vi "CMD_FIT.vi"(6 "Gantry in":refnum<class "Gantry Class.lvclass">, 8 "error in (no error)":errorcluster, 10 "Arguments":string[](array[string]), 11 "gScript Interpreter in":refnum<class "gScript Interpreter.lvclass">) -> (0 "error out":errorcluster, 3 "gScript Interpreter out":refnum<class "gScript Interpreter.lvclass">, 4 "Gantry out":refnum<class "Gantry Class.lvclass">)   [LabVIEW 2017, in "gScript Interpreter.lvclass"]
uses:
  gScript Interpreter.lvclass
  Shared Components/Gantry Class/Gantry Class.lvclass
  Shared Components/Vec3d Class/Vec3d Class.lvclass
  Shared Components/FlexWorktable/FlexWorktable.lvclass
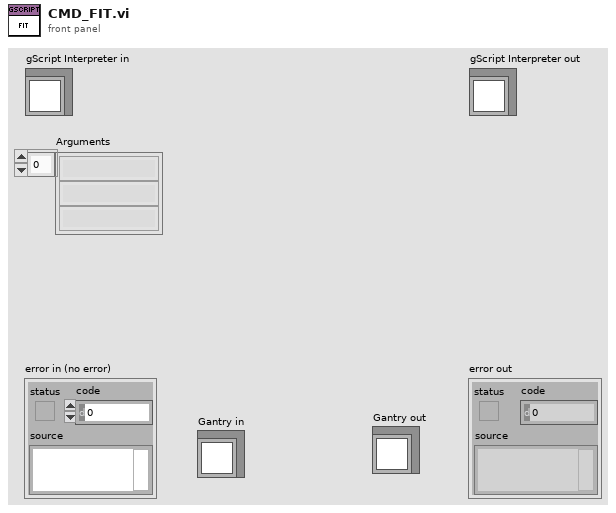
[diagram p1: front panel]
types:
  T1 = cluster{"fiducial location":refnum<class "Vec3d Class.lvclass">, "fiducial name":string}
  T2 = cluster{"Feature Coordinates":refnum<class "Vec3d Class.lvclass">, "Feature Name":string}[]
  T3 = typedef "Memory Cell.ctl" = cluster{"type":T4, "x":dbl, "y":dbl, "z":dbl, "w":dbl}
  T4 = typedef "Memory Cell Type Enum.ctl" = enum16{"integer", "float", "vector", "rotation"}
  T5 = cluster{"fiducial location":refnum<class "Vec3d Class.lvclass">, "fiducial name":string}[]
  T6 = typedef "Position_Orientation.ctl" = cluster{"Center":refnum<class "Vec3d Class.lvclass">, "Orientation":refnum<class "Orient3d Class.lvclass">}
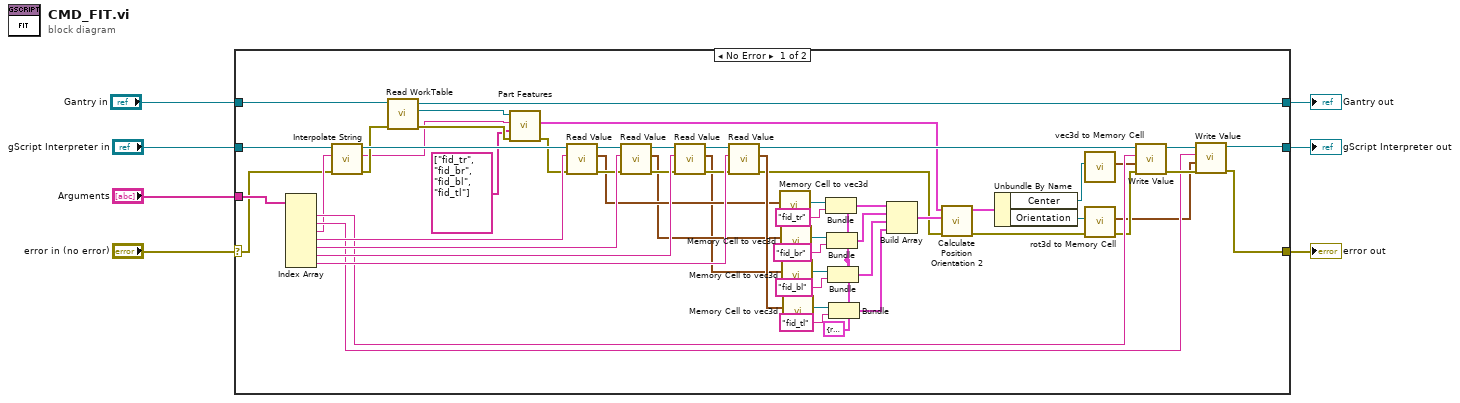
[diagram p0: block diagram]
diagram:
  n1 = case shown="No Error" "error in (no error)" {
    selector: "error in (no error)" -> [w16 w66]
    tunnel: [w19 w66] -> w6
    tunnel: [w20 w65] -> w4
    tunnel: "gScript Interpreter in" -> [w17 w65]
    tunnel: "Arguments" -> [w63 _]
    tunnel: "Gantry in" -> [w62 w64]
    tunnel: [w61 w64] -> w1
    frame No Error {
      w41 = T1 {"fiducial location"=refnum, "fiducial name"=""} ("fiducial with name")
      n2 = Index Array(array=w63) -> (element #1=w29:string, element #2=w23:string, element #3=w18:string, element #4=w60:string, element #5=w59:string, element #6=w58:string, element #7=w57:string)  [unwired: 7 in]
      n3 = call-dynamic "Interpolate String.vi"("error in (no error)"=w16, "Input String"=w18, "gScript Interpreter in"=w17) -> ("error out"=w14:errorcluster, "Output String"=w11:string, "gScript Interpreter out"=w15:refnum<class "gScript Interpreter.lvclass">)  [unwired: 6 in]
      n4 = call-dynamic "Read WorkTable.vi"("error in"=w14, "Gantry Class in"=w62) -> ("error out"=w12:errorcluster, "Worktable"=w13:refnum<class "FlexWorktable.lvclass">, "Gantry Class out"=w61:refnum<class "Gantry Class.lvclass">)  [unwired: 7 in]
      n5 = call-dynamic "Part Features.vi"("error in (no error)"=w12, "Feature Names"=string[] ["fid_tr", "fid_br", "fid_bl", "fid_tl"], "Part Name"=w11, "FlexWorktable in"=w13) -> ("error out"=w9:errorcluster, "Features"=w8:T2)  [unwired: 5 in, 1 out]
      n6 = call-dynamic "Read Value.vi"("error in (no error)"=w9, "String in"=w60, "gScript Interpreter in"=w15) -> ("error out"=w56:errorcluster, "Memory Cell"=w40:T3, "gScript Interpreter out"=w53:refnum<class "gScript Interpreter.lvclass">)  [unwired: 6 in]
      n7 = call-dynamic "Read Value.vi"("error in (no error)"=w56, "String in"=w59, "gScript Interpreter in"=w53) -> ("error out"=w55:errorcluster, "Memory Cell"=w39:T3, "gScript Interpreter out"=w52:refnum<class "gScript Interpreter.lvclass">)  [unwired: 6 in]
      n8 = call-dynamic "Read Value.vi"("error in (no error)"=w55, "String in"=w58, "gScript Interpreter in"=w52) -> ("error out"=w54:errorcluster, "Memory Cell"=w38:T3, "gScript Interpreter out"=w51:refnum<class "gScript Interpreter.lvclass">)  [unwired: 6 in]
      n9 = call-dynamic "Read Value.vi"("error in (no error)"=w54, "String in"=w57, "gScript Interpreter in"=w51) -> ("error out"=w32:errorcluster, "Memory Cell"=w50:T3, "gScript Interpreter out"=w30:refnum<class "gScript Interpreter.lvclass">)  [unwired: 6 in]
      n10 = call "Memory Cell to vec3d.vi"("Memory Cell"=w40) -> ("Vec3d out"=w43:refnum<class "Vec3d Class.lvclass">)  [unwired: 10 in]
      n11 = call "Memory Cell to vec3d.vi"("Memory Cell"=w39) -> ("Vec3d out"=w45:refnum<class "Vec3d Class.lvclass">)  [unwired: 10 in]
      n12 = call "Memory Cell to vec3d.vi"("Memory Cell"=w38) -> ("Vec3d out"=w47:refnum<class "Vec3d Class.lvclass">)  [unwired: 10 in]
      n13 = call "Memory Cell to vec3d.vi"("Memory Cell"=w50) -> ("Vec3d out"=w49:refnum<class "Vec3d Class.lvclass">)  [unwired: 10 in]
      n14 = Bundle(cluster=w41, "fiducial location"=w43, "fiducial name"="fid_tr") -> (w37:T1)
      n15 = Bundle(cluster=w41, "fiducial location"=w45, "fiducial name"="fid_br") -> (w36:T1)
      n16 = Bundle(cluster=w41, "fiducial location"=w47, "fiducial name"="fid_bl") -> (w35:T1)
      n17 = Bundle(cluster=w41, "fiducial location"=w49, "fiducial name"="fid_tl") -> (w34:T1)
      n18 = Build Array(w37, w36, w35, w34) -> (w33:T5)
      n19 = call "Calculate Position Orientation 2.vi"("error in"=w32, "Measured Global Positions"=w33, "Known Local Positions"=w8) -> ("error out"=w28:errorcluster, "PositionOrientation"=w31:T6)  [unwired: 6 in, 1 out]
      n20 = Unbundle By Name(w31) -> ("Center"=w27:refnum<class "Vec3d Class.lvclass">, "Orientation"=w22:refnum<class "Orient3d Class.lvclass">)
      n21 = call "vec3d to Memory Cell.vi"("Vec3d in"=w27) -> ("Memory Cell"=w26:T3)  [unwired: 10 in]
      n22 = call "rot3d to Memory Cell.vi"("Orient3d in"=w22) -> ("Memory Cell"=w21:T3)  [unwired: 10 in]
      n23 = call-dynamic "Write Value.vi"("error in (no error)"=w28, "Value"=w26, "Address"=w29, "gScript Interpreter in"=w30) -> ("error out"=w25:errorcluster, "gScript Interpreter out"=w24:refnum<class "gScript Interpreter.lvclass">)  [unwired: 6 in]
      n24 = call-dynamic "Write Value.vi"("error in (no error)"=w25, "Value"=w21, "Address"=w23, "gScript Interpreter in"=w24) -> ("error out"=w19:errorcluster, "gScript Interpreter out"=w20:refnum<class "gScript Interpreter.lvclass">)  [unwired: 6 in]
    }
    frame Error {
    }
  }
  "error out" <- w6
  "gScript Interpreter out" <- w4
  "Gantry out" <- w1
